vi "Build Endpoint.vi"(8 "error in (no error)":errorcluster, 9 "Port":u16, 10 "Address":string, 11 "RemoteControl.ZMQ in":refnum<class "RemoteControl.ZMQ.lvclass">) -> (0 "error out":errorcluster, 3 "RemoteControl.ZMQ out":refnum<class "RemoteControl.ZMQ.lvclass">)   [LabVIEW 2019, in "RemoteControl.ZMQ.lvlib" / "RemoteControl.ZMQ.lvclass"]
uses:
  RemoteControl.ZMQ.lvclass
  <vilib>/addons/zeromq/zeromq.lvlib
  <vilib>/addons/zeromq/endpoint_proto.ctl
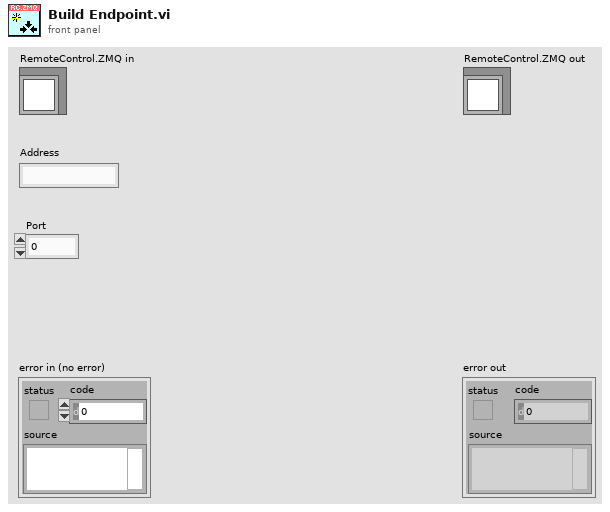
[diagram p1: front panel]
types:
  T1 = typedef "zeromq.lvlib/endpoint_proto.ctl" = enum16{"tcp", "udp", "inproc"}
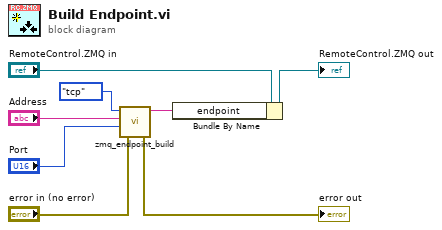
[diagram p0: block diagram]
diagram:
  n1 = call <vilib>:"zmq_endpoint_build.vi"("error in"="error in (no error)", "port"="Port", "address"="Address", "protocol (tcp)"=endpoint_proto."tcp") -> ("error out"=→"error out":errorcluster, "endpoint"=w2:string)  [unwired: 1 in, 1 out]
  n2 = Bundle By Name(cluster="RemoteControl.ZMQ in", "endpoint"=w2) -> (→"RemoteControl.ZMQ out":refnum<class "RemoteControl.ZMQ.lvclass">)
